vi "S&E Base string header.vi"(9 "error in (no error)":errorcluster, 13 "Delimiter(;)":string=";") -> (8 "Header":string, 10 "error out":errorcluster)   [LabVIEW 2010]
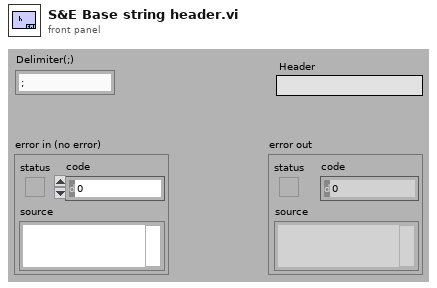
[diagram p1: front panel]
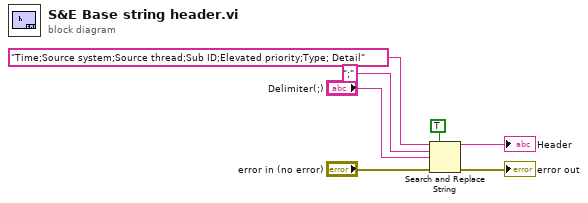
[diagram p0: block diagram]
diagram:
  n1 = Search and Replace String(replace all?=TRUE ("replace all? (F)"), input string="Time;Source system;Source thread;Sub ID;Elevated priority;Type; Detail" ("format string"), search string=";", replace string="Delimiter(;)", error in="error in (no error)") -> (result string=→"Header":string, error out=→"error out":errorcluster)  [unwired: 3 in, 2 out]
